vi "SetCurrGain.vi"(6 "time out":u32, 9 "Real1":dbl, 10 "类型":u32(ring)=4 items=["PCI5121"=1, "PCI9810"=2, "USBCAN1"=3, "USBCAN2"=4, "PCI9820"=5, "CAN232"=6, "PCI5110"=7, "CANLite(mini)"=8, "ISA9620"=9, "ISA5420"=10, "PC104CAN"=11, "CANET"=17, "DNP9810"=13, "USBCAN-E-U"=20, "USBCAN-2E-U"=21], 11 "Real2":dbl, 12 "设备索引":u32(ring) items=["0", "1", "2", "3", "4", "5", "6", "7", "8", "9", "10", "11", "12", "13", "14", "15", ""], 13 "AD1":u16, 15 "AD2":u16, 16 "CAN路数":u32(ring) items=["0", "1"]) -> (20 "set ok?":bool, 22 "Gain":u16)   [LabVIEW 2013]
uses:
  AutoBurn/Settings/ControlCAN.dll
panel:
  out "VCI_CAN_OBJ_T":T1 {"ID" format="%x"}
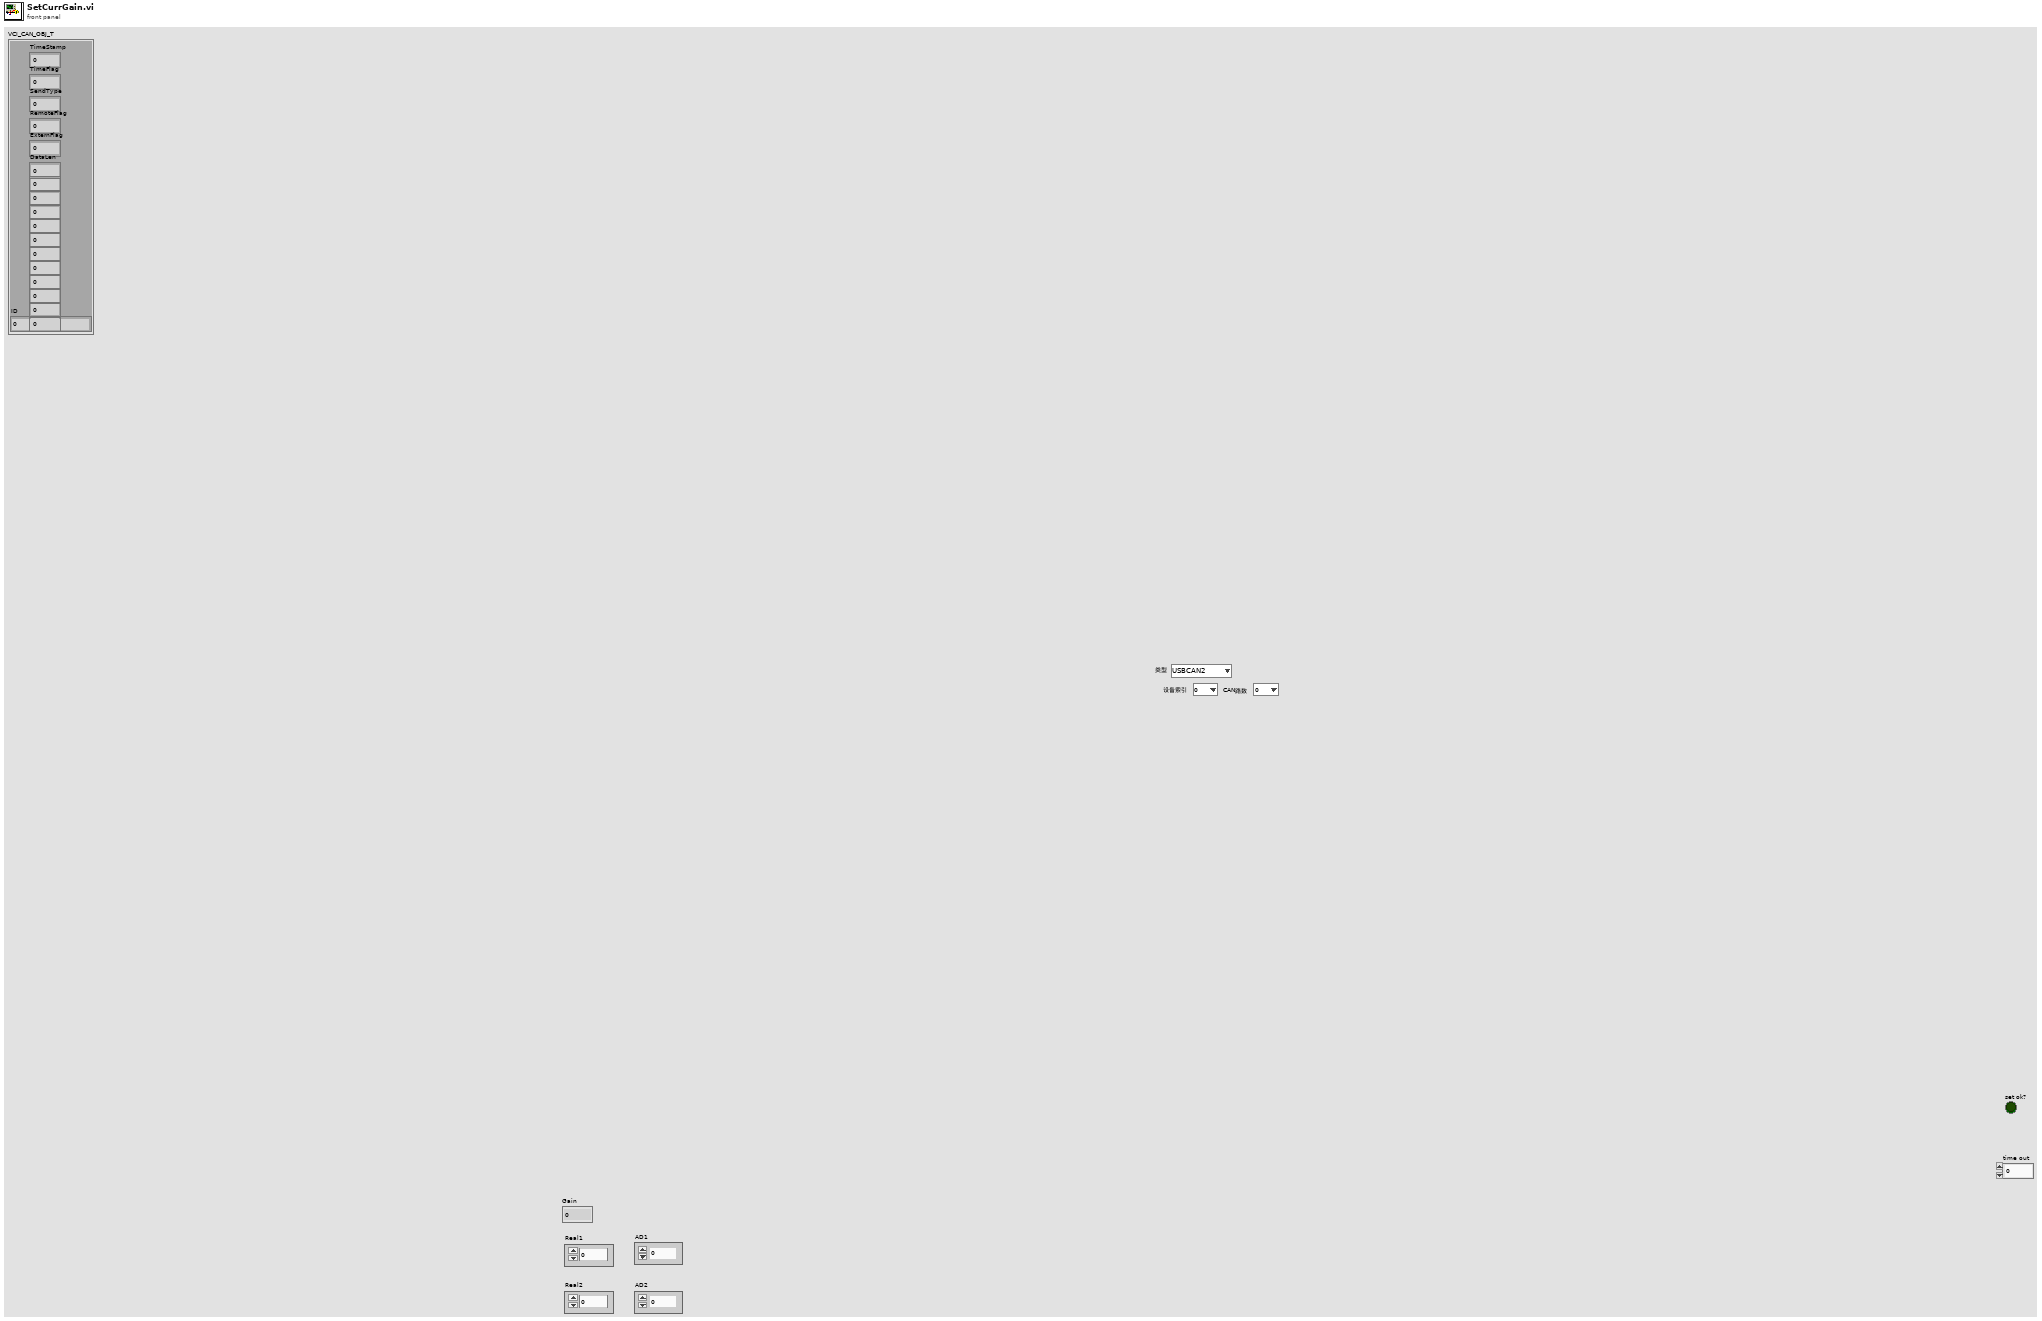
[diagram p1: front panel]
types:
  T1 = cluster{"ID":u32, "TimeStamp":u32, "TimeFlag":u8, "SendType":u8, "RemoteFlag":u8, "ExternFlag":u8, "DataLen":u8, u8, u8, u8, u8, u8, u8, u8, u8, u8, u8, u8}
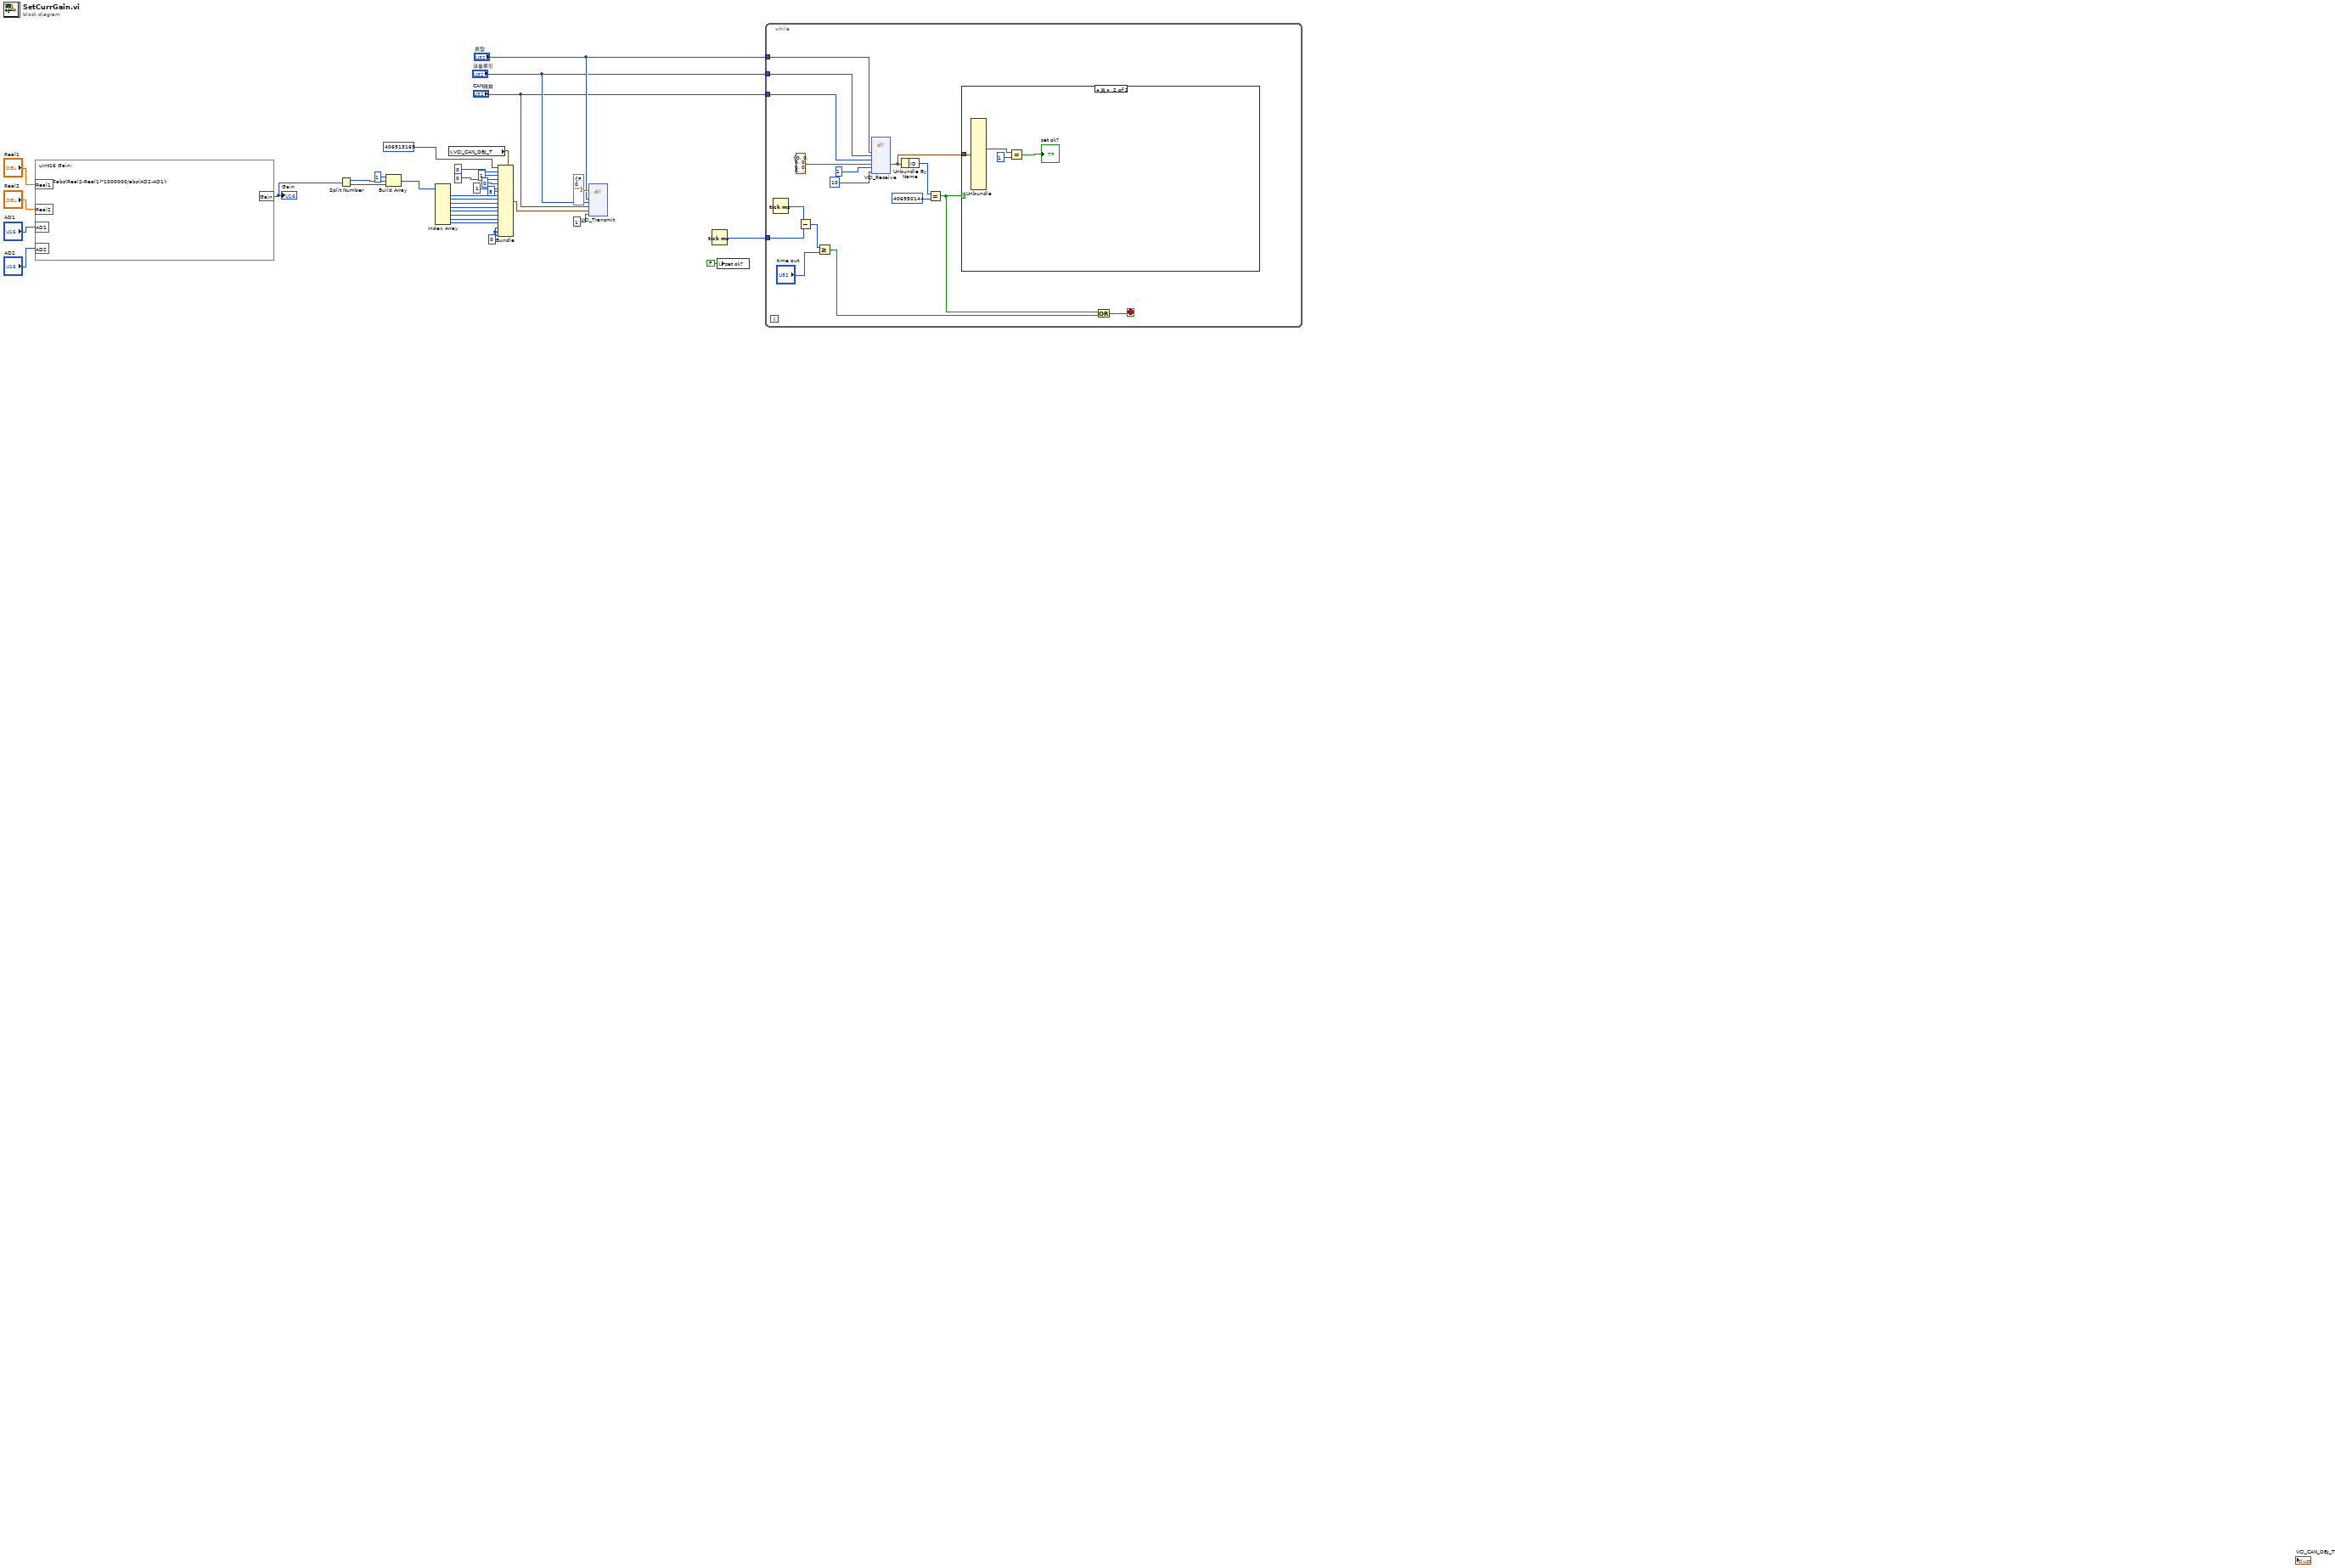
[diagram p0: block diagram]
diagram:
  w26 = u8 0 ("元素")
  n1 = formula code="uInt16 Gain;\n\n\nGain=abs(Real2-Real1)*1000000/abs(AD2-AD1);"("Real1"="Real1", "Real2"="Real2", "AD1"="AD1", "AD2"="AD2") -> ("Gain"=w5:u16)
  "Gain" <- w5
  n2 = Split Number(x=w5) -> (hi(x)=w4:u8, lo(x)=w3:u8)
  n3 = Build Array(u8 1 ("元素"), w4, w3) -> (w1:u8[])
  n4 = Index Array(array=w1) -> (element #1=w24:u8, element #2=w23:u8, element #3=w22:u8, element #4=w21:u8, element #5=w20:u8, element #6=w19:u8, element #7=w18:u8, element #8=w17:u8)  [unwired: 8 in]
  n5 = local read "VCI_CAN_OBJ_T"() -> (w30:T1)
  n6 = Bundle(cluster=w30, "ID"=u32 406913169 ("RemoteFlag"), "TimeStamp"=u8 0 ("RemoteFlag"), "TimeFlag"=u8 1, "SendType"=u8 0 ("DataLen"), "RemoteFlag"=u8 0, "ExternFlag"=u8 1, "DataLen"=u8 8, w24, w23, w22, w21, w20, w19, w18, w17, w26, w26, w26) -> (w31:T1)
  n7 = dll-call lib="F:/Bluewave New Energy/SVN_Work/AutoTest_TestStand/trunk/AutoTest_TestStand/Driver/ZlgCan/BHN01/AutoBurn/Settings/ControlCAN.dll" fn="VCI_Transmit"(error in=errorcluster {"status"=FALSE, "code"=0, "source"=""} ("错误输入（无错误）"), "DeviceType"="类型", "DeviceInd"="设备索引", "CANInd"="CAN路数", "pSend"=w31, "Len"=u32 1) -> ()  [unwired: 4 in, 6 out]
  n8 = Tick Count (ms)() -> (millisecond timer value=w34:u32)
  n9 = local write "set ok?"(FALSE ("x = y?")) -> ()
  n10 = while {
    tunnel: w34 -> [w46]
    tunnel: "类型" -> [w37]
    tunnel: "设备索引" -> [w36]
    tunnel: "CAN路数" -> [w35]
    stop <- w40 stop-if-true
    n11 = Tick Count (ms)() -> (millisecond timer value=w47:u32)
    n12 = Subtract(x=w47, y=w46) -> (x-y=w45:u32)
    n13 = Greater Or Equal?(x=w45, y="time out") -> (x >= y?=w41:bool)
    n14 = dll-call lib="F:/Bluewave New Energy/SVN_Work/AutoTest_TestStand/trunk/AutoTest_TestStand/Driver/ZlgCan/BHN01/AutoBurn/Settings/ControlCAN.dll" fn="VCI_Receive"("DeviceType"=w37, "DeviceInd"=w36, "CANInd"=w35, "pReceive"=T1 {"ID"=0, "TimeStamp"=0, "TimeFlag"=0, "SendType"=0, "RemoteFlag"=0, "ExternFlag"=0, "DataLen"=0, 0, 0, 0, 0, 0, 0, 0, 0, 0, 0, 0}, "Len"=u32 1, "WaitTime"=10) -> ("pReceive"=w39:T1)  [unwired: 8 in, 3 out]
    n15 = Unbundle By Name(w39) -> ("ID"=w43:u32)
    n16 = Equal?(x=w43, y=u32 406950144) -> (x = y?=w42:bool)
    n17 = case shown="真" w42 {
      tunnel: w39 -> [_ w54]
      frame False {
      }
      frame True {
        n18 = Unbundle(w54) -> (w51:u8)  [unwired: 17 out]
        n19 = Equal?(x=w51, y=u8 1) -> (x = y?=→"set ok?":bool)
      }
    }
    n20 = Or(x=w42, y=w41) -> (x .or. y?=w40:bool)
  }
